vi "Toolkit - Find All Clusters Target.vi"() -> ()   [LabVIEW 2017]
doc: "The target VI for the Toolkit - Find All Clusters example. Do NOT modify the contents of this VI. This is needed because alphabetizing within a running VI is not possible."
panel:
  out "Boolean":bool
  in  "String":string
  in  "Numeric":dbl
  in  "Control":T1
  # "Overview: The target VI for the Toolkit - Find All Clusters example\nInstructions:\n1. Do not modify or remove\n\nThis is needed for finding all clusters using VI scripting and the ACE toolkit."
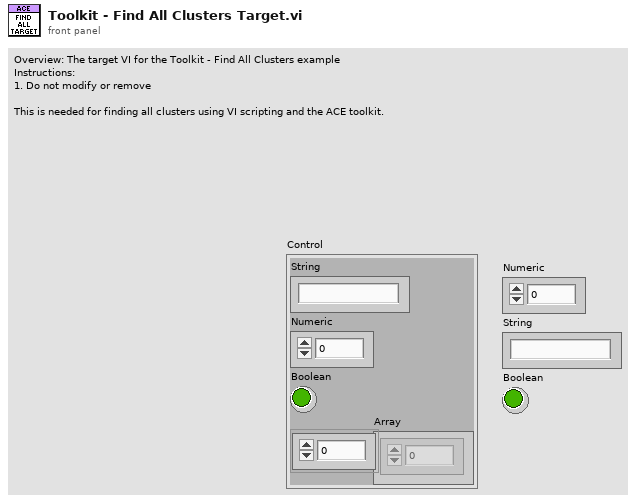
[diagram p1: front panel]
types:
  T1 = cluster{"String":string, "Numeric":dbl, "Boolean":bool, "Array":dbl[]}
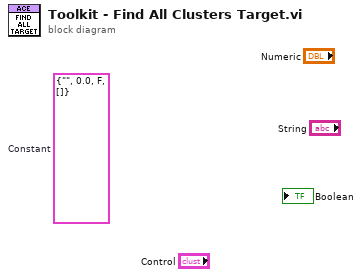
[diagram p0: block diagram]
diagram:
  (unwired) T1 {"String"="", "Numeric"=0.0, "Boolean"=FALSE, "Array"=[]}  # Constant
